vi "test8-AsyncMessageWithoutReply_API.vi"(8 "error in (no error)":errorcluster, 11 "TestCase in":refnum<class "testcase-CSMMessage.lvclass">) -> (0 "error out":errorcluster, 3 "TestCase out":refnum<class "testcase-CSMMessage.lvclass">)   [LabVIEW 2017, in "testcase-CSMMessage.lvclass"]
uses:
  testcase-CSMMessage.lvclass
  7412589e-de49-4983-aece-358686b48526.vi
  <vilib>/addons/_JKI Toolkits/VI Tester/TestCase.llb/TestCase.lvclass
  src/user.lib/_NEVSTOP/Communicable State Machine(CSM)/Communicable State Machine.lvlib
  C:/Program Files (x86)/National Instruments/LabVIEW 2017/vi.lib/addons/_JKI Toolkits/VI Tester/TestCase.llb/TestCase.lvclass
panel:
  out "Loop count":i32
  out "concatenated string":string
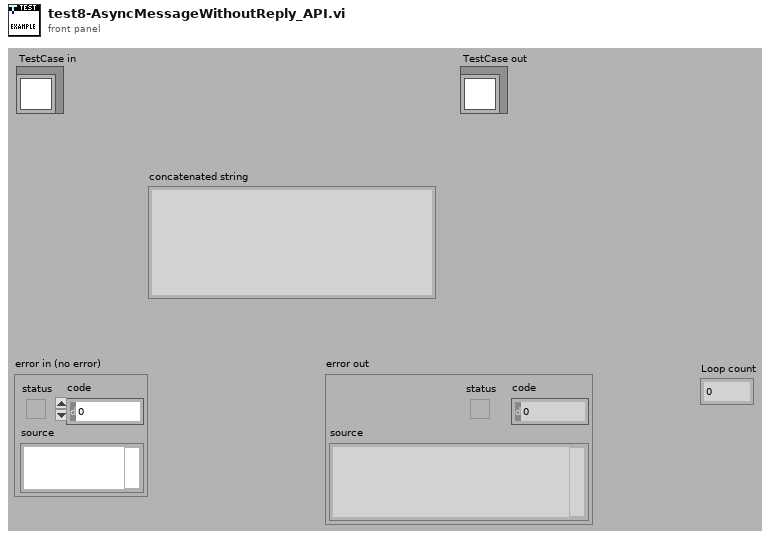
[diagram p1: front panel]
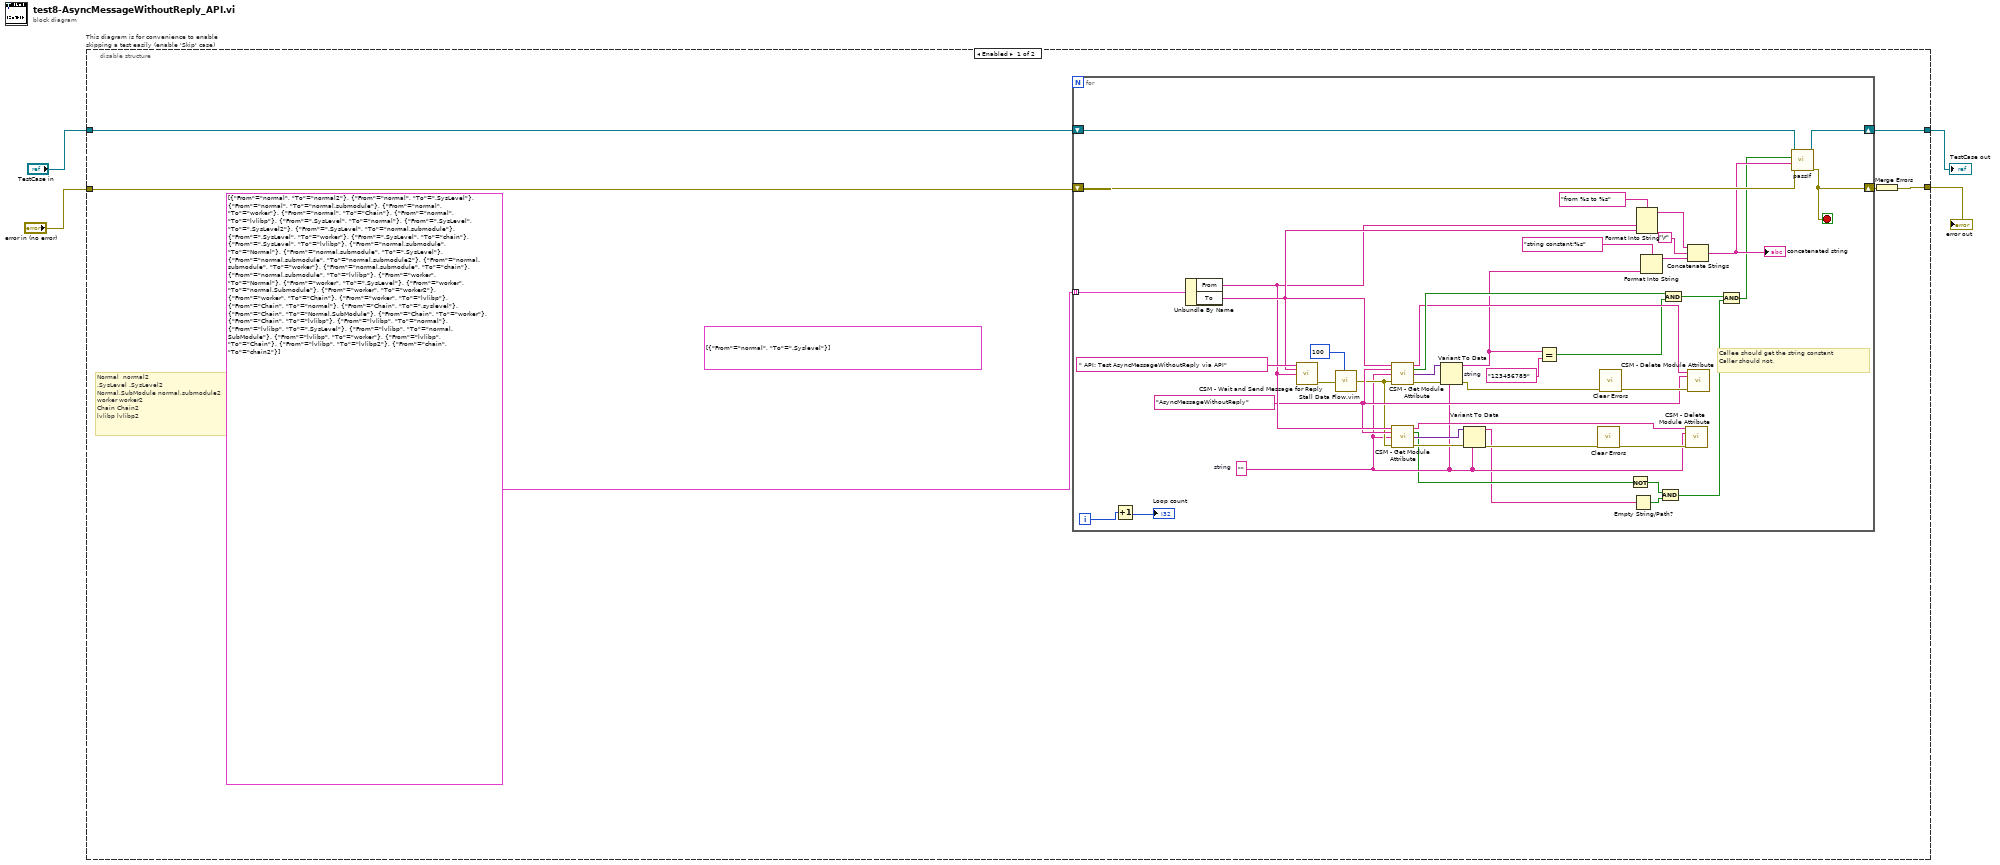
[diagram p0: block diagram]
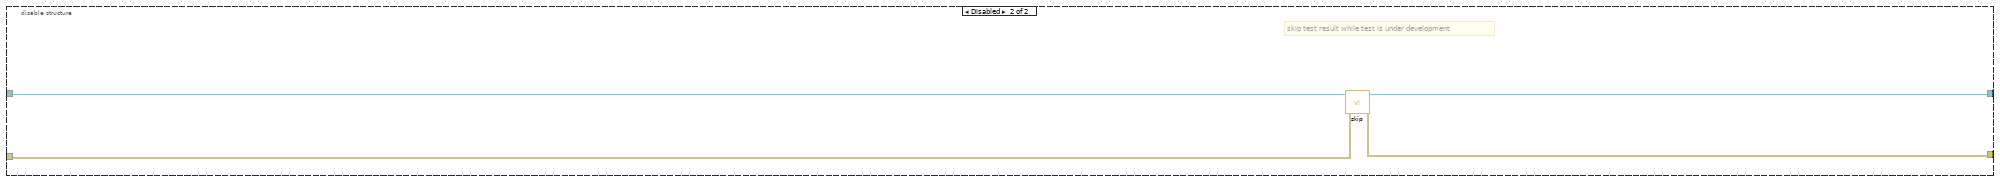
[diagram p2: hidden frame]
diagram:
  n1 = disable-structure "This diagram is for convenience to enable skipping a test easily (enable 'Skip' case)" shown="Enabled" {
    disable-tunnel: "TestCase in" -> [w10 w56]
    disable-tunnel: [w9 w54] -> w1
    disable-tunnel: [w6 w55] -> w3
    disable-tunnel: "error in (no error)" -> [w7 w53]
    frame Enabled {
      (unwired) cluster{"From":string, "To":string}[] [{"From"="normal", "To"=".Syslevel"}]
      # "Normal  normal2\n.SysLevel .SysLevel2\nNormal.SubModule normal.submodule2\nworker worker2\nChain Chain2\nlvlibp lvlibp2"
      n2 = for {
        tunnel: cluster{"From":string, "To":string}[] [{"From"="normal", "To"="normal2"}, {"From"="normal", "To"=".SysLevel"}, {"From"="normal", "To"="normal.submodule"}, {"From"="normal", "To"="worker"}, {"From"="normal", "To"="Chain"}, {"From"="normal", "To"="lvlibp"}, {"From"=".SysLevel", "To"="normal"}, {"From"=".SysLevel", "To"=".SysLevel2"}, {"From"=".SysLevel", "To"="normal.submodule"}, {"From"=".SysLevel", "To"="worker"}, {"From"=".SysLevel", "To"="chain"}, {"From"=".SysLevel", "To"="lvlibp"}, {"From"="normal.submodule", "To"="Normal"}, {"From"="normal.submodule", "To"=".SysLevel"}, {"From"="normal.submodule", "To"="normal.submodule2"}, {"From"="normal.submodule", "To"="worker"}, {"From"="normal.submodule", "To"="chain"}, {"From"="normal.submodule", "To"="lvlibp"}, {"From"="worker", "To"="Normal"}, {"From"="worker", "To"=".SysLevel"}, {"From"="worker", "To"="normal.Submodule"}, {"From"="worker", "To"="worker2"}, {"From"="worker", "To"="Chain"}, {"From"="worker", "To"="lvlibp"}, {"From"="Chain", "To"="normal"}, {"From"="Chain", "To"=".syslevel"}, {"From"="Chain", "To"="Normal.SubModule"}, {"From"="Chain", "To"="worker"}, {"From"="Chain", "To"="lvlibp"}, {"From"="lvlibp", "To"="normal"}, {"From"="lvlibp", "To"=".SysLevel"}, {"From"="lvlibp", "To"="normal.SubModule"}, {"From"="lvlibp", "To"="worker"}, {"From"="lvlibp", "To"="Chain"}, {"From"="lvlibp", "To"="lvlibp2"}, {"From"="chain", "To"="chain2"}] -> [w45] mode=indexing
        shift-right: [w51] -> w9
        shift-left: w10 -> [w52]
        shift-right: [w35] -> w8
        shift-left: w7 -> [w50]
        i -> [w14]
        stop <- w35 stop-if-true
        w32 = "123456789"  # string
        w22 = ""  # string
        w29 = "AsyncMessageWithoutReply" ("State With Arguments")
        # "Callee should get the string constant\nCaller should not."
        n3 = Increment(x=w14) -> (x+1=→"Loop count":i32)
        n4 = Unbundle By Name(w45) -> ("From"=w30:string, "To"=w34:string)
        n5 = call "CSM - Wait and Send Message for Reply.vi"("State"=" API: Test AsyncMessageWithoutReply via API", "Arguments (\"\")"=w34, "Target Module"=w30) -> ("error out"=w12:errorcluster)  [unwired: 10 in, 2 out]
        n6 = call "Stall Data Flow.vim"("value in"=w12, "milliseconds to wait"=u32 100) -> ("value out"=w28:errorcluster)  [unwired: 1 out]
        n7 = call "CSM - Get Module Attribute.vi"("CSM Name"=w34, "Attribute"=w29, "Default Value (Empty Variant)"=w22, "Error In"=w28) -> ("CSM Name (Dup)"=w43:string, "Found"=w46:bool, "Value"=w47:variant, "error out"=w48:errorcluster)  [unwired: 7 in, 1 out]
        n8 = call "CSM - Get Module Attribute.vi"("CSM Name"=w30, "Attribute"=w29, "Default Value (Empty Variant)"=w22, "Error In"=w28) -> ("CSM Name (Dup)"=w23:string, "Found"=w21:bool, "Value"=w24:variant, "error out"=w27:errorcluster)  [unwired: 7 in, 1 out]
        n9 = Variant To Data(error in=w48, type=w22, Variant=w47) -> (data=w31:string, error out=w37:errorcluster)
        n10 = Variant To Data(error in=w27, type=w22, Variant=w24) -> (data=w20:string, error out=w26:errorcluster)
        n11 = Equal?(x=w31, y=w32) -> (x = y?=w33:bool)
        n12 = call <vilib>:"Clear Errors.vi"("error in (no error)"=w26) -> ("error out"=w25:errorcluster)  [unwired: 5 in, 1 out]
        n13 = call <vilib>:"Clear Errors.vi"("error in (no error)"=w37) -> ("error out"=w36:errorcluster)  [unwired: 5 in, 1 out]
        n14 = Not(x=w21) -> (.not. x?=w17:bool)
        n15 = Empty String/Path?(string/path=w20) -> (empty?=w19:bool)
        n16 = Format Into String(format string="from %s to %s", w30, w34) -> (resulting string=w39:string)  [unwired: 2 in, 1 out]
        n17 = Format Into String(format string="string constant:%s", w31) -> (resulting string=w42:string)  [unwired: 2 in, 1 out]
        n18 = And(x=w17, y=w19) -> (x .and. y?=w15:bool)
        n19 = And(x=w46, y=w33) -> (x .and. y?=w18:bool)
        n20 = call "CSM - Delete Module Attribute.vi"("CSM Name"=w23, "Attribute"=w22, "Error In"=w25) -> ()  [unwired: 9 in, 4 out]
        n21 = Concatenate Strings(w39, "\r", w42) -> (w40:string)
        "concatenated string" <- w40
        n22 = call "CSM - Delete Module Attribute.vi"("CSM Name"=w43, "Attribute"=w29, "Error In"=w36) -> ()  [unwired: 9 in, 4 out]
        n23 = And(x=w18, y=w15) -> (x .and. y?=w16:bool)
        n24 = call-dynamic "passIf.vi"("error in (no error)"=w50, "message (\"\")"=w40, "pass"=w16, "TestCase in"=w52) -> ("error out"=w35:errorcluster, "TestCase out"=w51:refnum<class "testcase-CSMMessage.lvclass">)  [unwired: 6 in]
      }
      n25 = Merge Errors(w8) -> (w6:errorcluster)
    }
    frame Disabled {
      # "skip test result while test is under development"
      n26 = call <vilib>:"skip.vi"("error in (no error)"=w53, "TestCase in"=w56) -> ("error out"=w55:errorcluster, "TestCase out"=w54:refnum<class "testcase-CSMMessage.lvclass">)  [unwired: 8 in]
    }
  }
  "error out" <- w3
  "TestCase out" <- w1
